vi "range.vi"(9 "Value":dbl, 10 "lower limit":dbl, 11 "upper limit":dbl) -> (3 "In range?":bool)   [LabVIEW 2015]
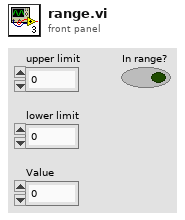
[diagram p1: front panel]
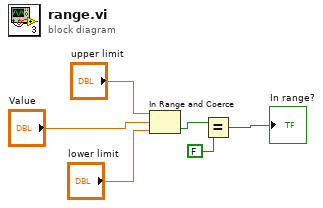
[diagram p0: block diagram]
diagram:
  n1 = In Range and Coerce(upper limit="upper limit", x="Value", lower limit="lower limit") -> (In Range?=w3:bool)  [unwired: 1 out]
  n2 = Equal?(x=w3, y=FALSE) -> (x = y?=→"In range?":bool)
